vi "x-axis.vi"(8 "error in (no error)":errorcluster, 11 "Varian Magnet Scan in":refnum<class "Varian Magnet Scan.lvclass">) -> (0 "error out":errorcluster, 1 "Label":string, 2 "Unit":string, 3 "Varian Magnet Scan out":refnum<class "Varian Magnet Scan.lvclass">)   [LabVIEW 2009, in "Varian Magnet Scan.lvclass"]
uses:
  Varian Magnet Scan.lvclass
  Scanner/Scanner.lvclass
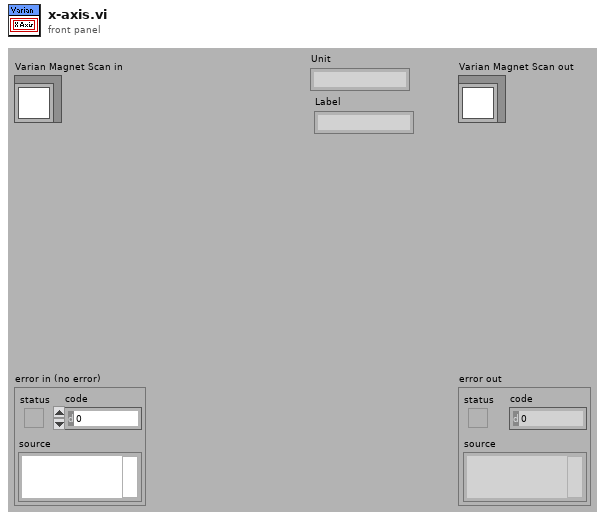
[diagram p1: front panel]
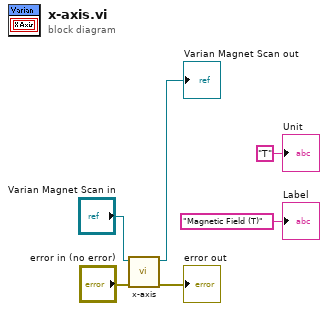
[diagram p0: block diagram]
diagram:
  n1 = call-parent "x-axis.vi"("error in (no error)"="error in (no error)", "Scanner in"="Varian Magnet Scan in") -> ("error out"=→"error out":errorcluster, "Scanner out"=→"Varian Magnet Scan out":refnum<class "Varian Magnet Scan.lvclass">)  [unwired: 6 in, 2 out]
  "Label" <- "Magnetic Field (T)" ("Label")
  "Unit" <- "T" ("Unit")
